vi "AIM664 Read BSP Version.vi"() -> ()   [LabVIEW 2020]
uses:
  AIM664LV.lvlib
panel:
  out "NuOfResources":u32
  out "error out":errorcluster
  out "BSP Special Version Out":T1
  out "output BSP Version":T2
  in  "Client & Server":T3={"SrvName"="local", "ClHostName"="local", "ClUser"="Brett", "ClApplication"="Test", "ClApplicationVersion"="V01.00", "ResourceID"=1, "Privileges"=4294967295} {"Privileges" min=4294967295 format="%x"}
  out "NuOfServers":u32
  # "ARINC 664 Read BSP Version"
  # "Overview: Queries the boards available in a system and present some properties of those resources.\nRequirement: At least one AIM ARINC-664 board with installed AIM ARINC 664 BSP.\nRestrictions: None.\nInstruction:\n1. Run the VI.\n2. Verify the resources available. If no error is presented, you will see all of the resources in the Resources."
  # "FdxCntSrvResrcCvi\nFdxLoginCvi"
  # "FdxInitCvi"
  # "FdxReadBSPVersionCvi"
  # "FdxReadBSPVersionSpecialCvi"
  # "FdxLogoutCvi"
  # "Input"
  # "Input"
  # "Input"
  # "Input"
  # "Output"
  # "Output"
  # "Output"
  # "Output"
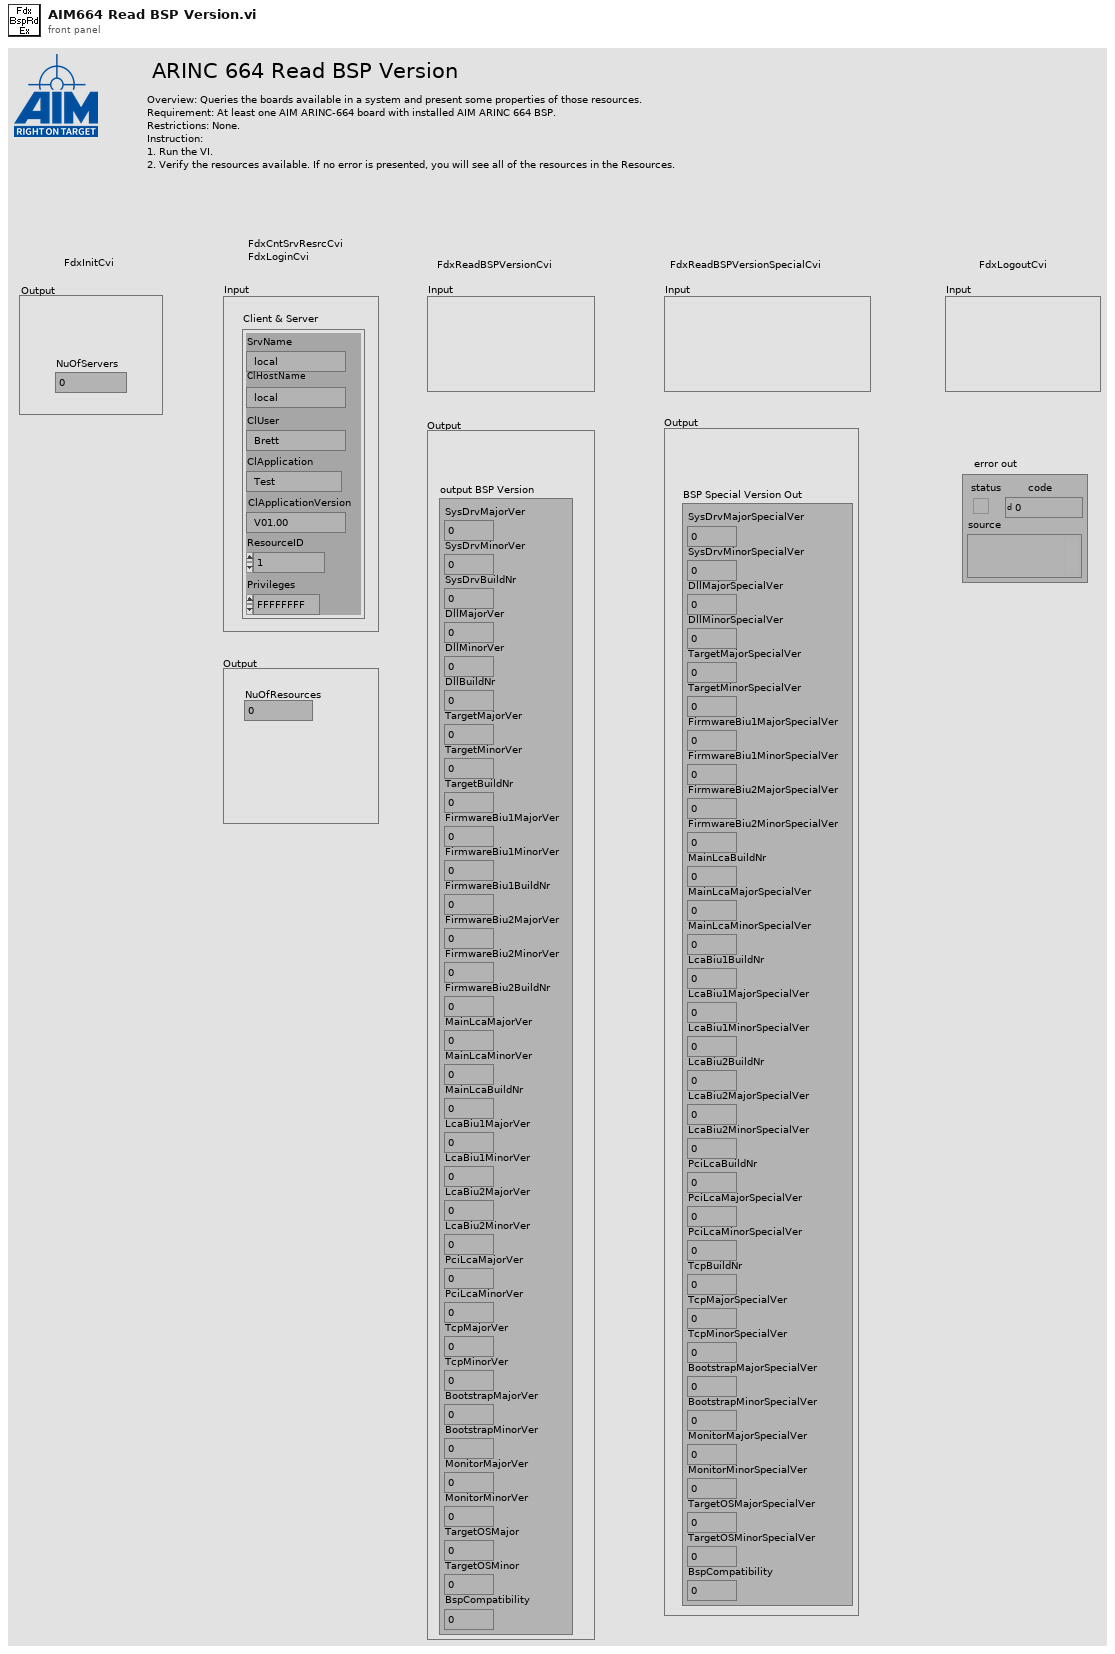
[diagram p1: front panel]
types:
  T1 = cluster{"SysDrvMajorSpecialVer":u32, "SysDrvMinorSpecialVer":u32, "DllMajorSpecialVer":u32, "DllMinorSpecialVer":u32, "TargetMajorSpecialVer":u32, "TargetMinorSpecialVer":u32, "FirmwareBiu1MajorSpecialVer":u32, "FirmwareBiu1MinorSpecialVer":u32, "FirmwareBiu2MajorSpecialVer":u32, "FirmwareBiu2MinorSpecialVer":u32, "MainLcaBuildNr":u32, "MainLcaMajorSpecialVer":u32, "MainLcaMinorSpecialVer":u32, "LcaBiu1BuildNr":u32, "LcaBiu1MajorSpecialVer":u32, "LcaBiu1MinorSpecialVer":u32, "LcaBiu2BuildNr":u32, "LcaBiu2MajorSpecialVer":u32, "LcaBiu2MinorSpecialVer":u32, "PciLcaBuildNr":u32, "PciLcaMajorSpecialVer":u32, "PciLcaMinorSpecialVer":u32, "TcpBuildNr":u32, "TcpMajorSpecialVer":u32, "TcpMinorSpecialVer":u32, "BootstrapMajorSpecialVer":u32, "BootstrapMinorSpecialVer":u32, "MonitorMajorSpecialVer":u32, "MonitorMinorSpecialVer":u32, "TargetOSMajorSpecialVer":u32, "TargetOSMinorSpecialVer":u32, "BspCompatibility":u32}
  T2 = cluster{"SysDrvMajorVer":u32, "SysDrvMinorVer":u32, "SysDrvBuildNr":u32, "DllMajorVer":u32, "DllMinorVer":u32, "DllBuildNr":u32, "TargetMajorVer":u32, "TargetMinorVer":u32, "TargetBuildNr":u32, "FirmwareBiu1MajorVer":u32, "FirmwareBiu1MinorVer":u32, "FirmwareBiu1BuildNr":u32, "FirmwareBiu2MajorVer":u32, "FirmwareBiu2MinorVer":u32, "FirmwareBiu2BuildNr":u32, "MainLcaMajorVer":u32, "MainLcaMinorVer":u32, "MainLcaBuildNr":u32, "LcaBiu1MajorVer":u32, "LcaBiu1MinorVer":u32, "LcaBiu2MajorVer":u32, "LcaBiu2MinorVer":u32, "PciLcaMajorVer":u32, "PciLcaMinorVer":u32, "TcpMajorVer":u32, "TcpMinorVer":u32, "BootstrapMajorVer":u32, "BootstrapMinorVer":u32, "MonitorMajorVer":u32, "MonitorMinorVer":u32, "TargetOSMajor":u32, "TargetOSMinor":u32, "BspCompatibility":u32}
  T3 = cluster{"SrvName":string, "ClHostName":string, "ClUser":string, "ClApplication":string, "ClApplicationVersion":string, "ResourceID":u32, "Privileges":u32}
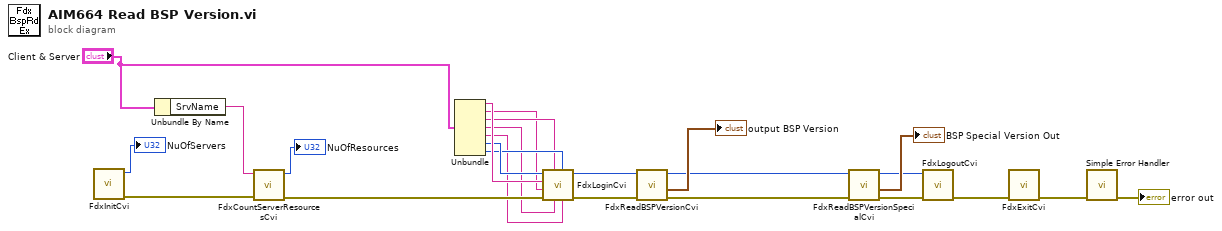
[diagram p0: block diagram]
diagram:
  n1 = call "FdxInitCvi.vi"() -> ("error out"=w20:errorcluster, "Number of Servers"=→"NuOfServers":u32)  [unwired: 10 in]
  n2 = Unbundle By Name("Client & Server") -> ("SrvName"=w16:string)
  n3 = call "FdxCountServerResourcesCvi.vi"("error in"=w20, "SrvName (local)"=w16) -> ("error out"=w19:errorcluster, "Number of Resources"=→"NuOfResources":u32)  [unwired: 8 in]
  n4 = Unbundle("Client & Server") -> ("SrvName"=w9:string, "ClHostName"=w5:string, "ClUser"=w6:string, "ClApplication"=w4:string, "ClApplicationVersion"=w3:string, "ResourceID"=w8:u32, "Privileges"=w7:u32)
  n5 = call "FdxLoginCvi.vi"("ClApplicationVersion"=w3, "Privileges"=w7, "ClApplication"=w4, "ClUser"=w6, "error in"=w19, "ClHostName"=w5, "SrvName"=w9, "ResourceID"=w8) -> ("error out"=w24:errorcluster, "InstrumentHandle"=w13:u32)  [unwired: 2 in]
  n6 = call "FdxReadBSPVersionCvi.vi"("error in"=w24, "InstrumentHandle_board in"=w13) -> ("error out"=w23:errorcluster, "BSP Version Out"=→"output BSP Version":T2, "InstrumentHandle_board out"=w12:u32)  [unwired: 7 in]
  n7 = call "FdxReadBSPVersionSpecialCvi.vi"("error in"=w23, "InstrumentHandle_board in"=w12) -> ("error out"=w22:errorcluster, "BSP Special Version Out"=→"BSP Special Version Out":T1, "InstrumentHandle_board out"=w11:u32)  [unwired: 7 in]
  n8 = call "FdxLogoutCvi.vi"("error in"=w22, "InstrumentHandle"=w11) -> ("error out"=w21:errorcluster)  [unwired: 9 in]
  n9 = call "FdxExitCvi.vi"("error in"=w21) -> ("error out"=w2:errorcluster)  [unwired: 10 in]
  n10 = call <vilib>:"Simple Error Handler.vi"("error in (no error)"=w2) -> ("error out"=→"error out":errorcluster)  [unwired: 4 in, 4 out]
